vi "Pic Plot Cross.vi"(6 "Color":u32(colorbox)=6618880, 8 "error in (no error)":errorcluster, 9 "Line":cluster{"Size":i32, "Width":u16}={"Size"=3, "Width"=1}, 10 "Position":cluster{"Centerx":i32, "Centery":i32}, 11 "Picture in":picture) -> (0 "error out":errorcluster, 3 "Picture out":picture)   [LabVIEW 2018, in "Picture Process.lvclass"]
uses:
  Picture Process.lvclass
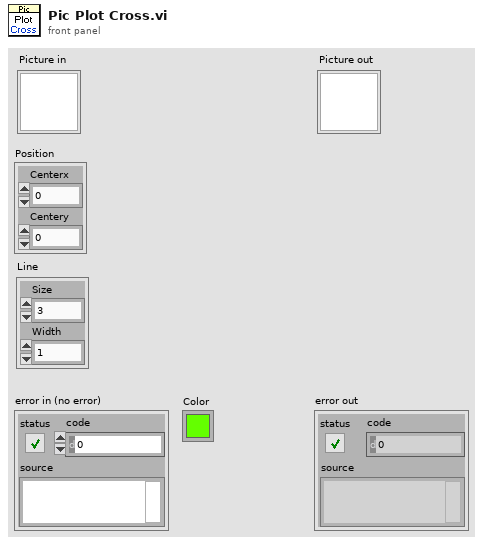
[diagram p1: front panel]
types:
  T1 = cluster{"Width":u16, "Style":enum32{"Solid", "Dash", "Dot", "DashDot", "DashDotDot"}}
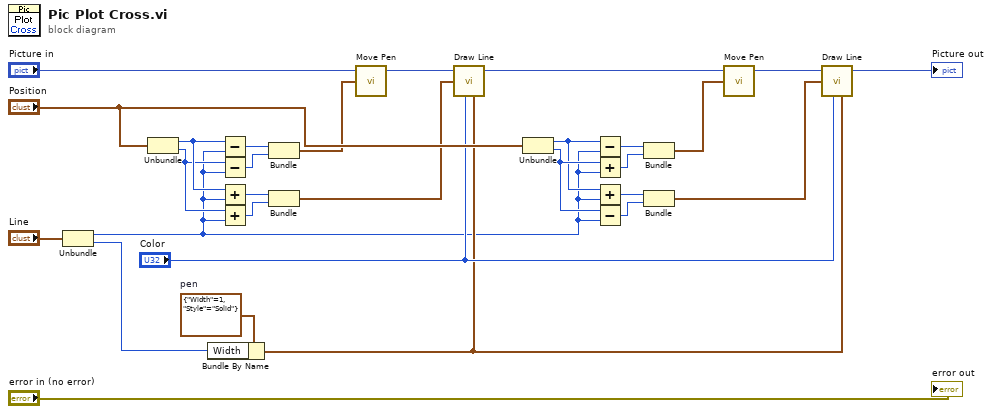
[diagram p0: block diagram]
diagram:
  w13 = T1 {"Width"=1, "Style"=enum."Solid"}  # pen
  n1 = Unbundle("Line") -> ("Size"=w2:i32, "Width"=w1:u16)
  n2 = Unbundle("Position") -> ("Centerx"=w24:i32, "Centery"=w23:i32)
  n3 = Bundle By Name(cluster=w13, "Width"=w1) -> (w6:T1)
  n4 = Subtract(x=w24, y=w2) -> (x-y=w28:i32)
  n5 = Subtract(x=w23, y=w2) -> (x-y=w27:i32)
  n6 = Add(x=w24, y=w2) -> (x+y=w25:i32)
  n7 = Add(x=w23, y=w2) -> (x+y=w26:i32)
  n8 = Bundle(w28, w27) -> (w10:cluster{i32, i32})  [unwired: 1 in]
  n9 = Bundle(w25, w26) -> (w14:cluster{i32, i32})  [unwired: 1 in]
  n10 = call <vilib>:"Move Pen.vi"("new position"=w10, "picture"="Picture in") -> ("new picture"=w16:picture)  [unwired: 3 in]
  n11 = call <vilib>:"Draw Line.vi"("picture"=w16, "end point"=w14, "color(black)"="Color", "pen"=w6) -> ("new picture"=w11:picture)  [unwired: 5 in]
  n12 = Unbundle("Position") -> ("Centerx"=w21:i32, "Centery"=w22:i32)
  n13 = Subtract(x=w21, y=w2) -> (x-y=w17:i32)
  n14 = Add(x=w22, y=w2) -> (x+y=w18:i32)
  n15 = Add(x=w21, y=w2) -> (x+y=w20:i32)
  n16 = Subtract(x=w22, y=w2) -> (x-y=w19:i32)
  n17 = Bundle(w17, w18) -> (w9:cluster{i32, i32})  [unwired: 1 in]
  n18 = Bundle(w20, w19) -> (w8:cluster{i32, i32})  [unwired: 1 in]
  n19 = call <vilib>:"Move Pen.vi"("new position"=w9, "picture"=w11) -> ("new picture"=w12:picture)  [unwired: 3 in]
  n20 = call <vilib>:"Draw Line.vi"("picture"=w12, "end point"=w8, "color(black)"="Color", "pen"=w6) -> ("new picture"=→"Picture out":picture)  [unwired: 5 in]
  "error out" <- "error in (no error)"
